vi "Parametros.vi"(0 "VetorDeDados":dbl[][](array[numeric]), 7 "area":dbl, 9 "irradiancia":dbl, 11 "pontos":dbl) -> (3 "FF":dbl, 4 "Icc":dbl, 6 "Vca":dbl, 8 "Pmp":dbl, 10 "Vmp":dbl, 14 "eficiencia":dbl, 15 "Imp":dbl)   [LabVIEW 2012]
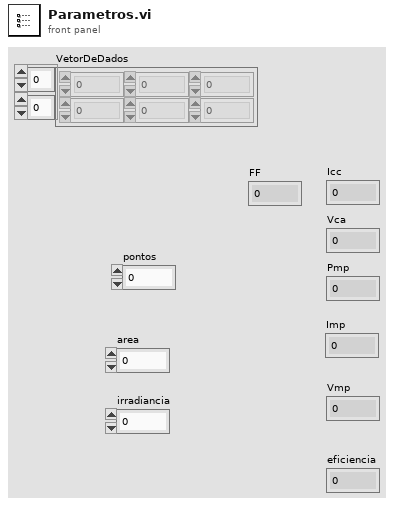
[diagram p1: front panel]
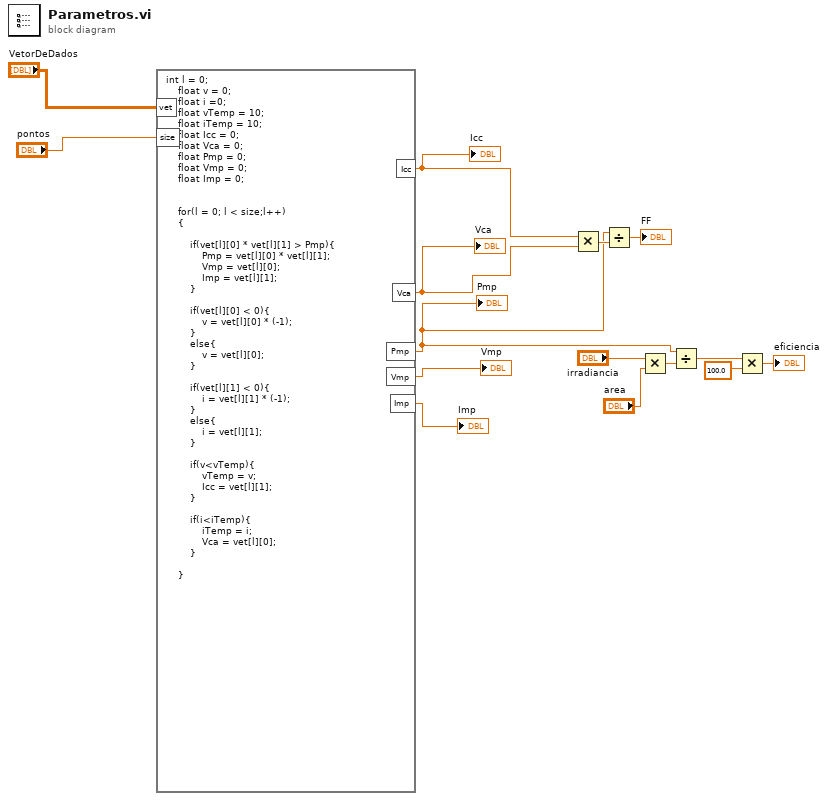
[diagram p0: block diagram]
diagram:
  n1 = formula code="int l = 0;\n    float v = 0;\n    float i =0;\n    float vTemp = 10;\n    float iTemp = 10;\n    float Icc = 0;\n    float Vca = 0;\n    float Pmp = 0;\n    float Vmp = 0;\n    float Imp = 0;\n\n\n    for(l = 0; l < size;l++)\n    {\n    \n        if(vet[l][0] * vet[l][1] > Pmp){\n            Pmp = vet[l][0] * vet[l][1];\n            Vmp = vet[l][0];\n            Imp = vet[l][1];\n        }\n\n        if(vet[l][0] < 0){\n            v = vet[l][0] * (-1);\n        }\n        else{\n            v = vet[l][0];\n        }\n\n        if(vet[l][1] < 0){\n            i = vet[l][1] * (-1);\n        }\n        else{\n            i = vet[l][1];\n        }\n\n        if(v<vTemp){\n            vTemp = v;\n            Icc = vet[l][1];\n        }\n\n        if(i<iTemp){\n            iTemp = i;\n            Vca = vet[l][0];\n        }\n\n    }"("vet"="VetorDeDados", "size"="pontos") -> ("Icc"=w5:dbl, "Vca"=w4:dbl, "Pmp"=w2:dbl, "Imp"=→"Imp":dbl, "Vmp"=→"Vmp":dbl)
  "Vca" <- w4
  "Pmp" <- w2
  "Icc" <- w5
  n2 = Multiply(x=w5, y=w4) -> (x*y=w3:dbl)
  n3 = Divide(x=w2, y=w3) -> (x/y=→"FF":dbl)
  n4 = Multiply(x="irradiancia", y="area") -> (x*y=w9:dbl)
  n5 = Divide(x=w2, y=w9) -> (x/y=w8:dbl)
  n6 = Multiply(x=w8, y=100.0) -> (x*y=→"eficiencia":dbl)
